vi "UpdateData.vi"(6 "Products":string[](array[string]), 8 "error in (no error)":errorcluster, 9 "Prices":dbl[](array[numeric]), 10 "Stock":i32[](array[numeric]), 11 "Prooduct Actor in":refnum<class "Prooduct Actor.lvclass">) -> (0 "error out":errorcluster, 3 "Prooduct Actor out":refnum<class "Prooduct Actor.lvclass">)   [LabVIEW 2020, in "Prooduct Actor.lvlib" / "Prooduct Actor.lvclass"]
uses:
  Prooduct Actor.lvclass
  Prooduct Actor.lvclass/Prooduct Actor.ctl
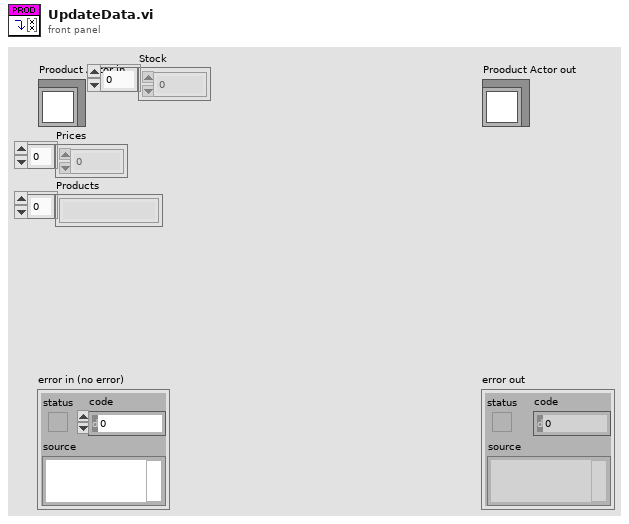
[diagram p1: front panel]
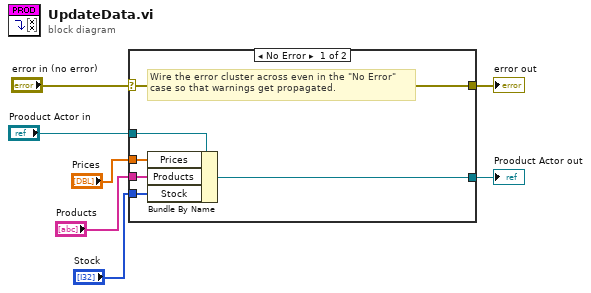
[diagram p0: block diagram]
diagram:
  n1 = case shown="No Error" "error in (no error)" {
    selector: "error in (no error)" -> [w13 w15]
    tunnel: [w13 w15] -> w6
    tunnel: [w11 w14] -> w4
    tunnel: "Prooduct Actor in" -> [w12 w14]
    tunnel: "Stock" -> [w10 _]
    tunnel: "Products" -> [w9 _]
    tunnel: "Prices" -> [w8 _]
    frame No Error {
      # "Wire the error cluster across even in the \"No Error\"\ncase so that warnings get propagated."
      n2 = Bundle By Name(cluster=w12, "Prices"=w8, "Products"=w9, "Stock"=w10) -> (w11:refnum<class "Prooduct Actor.lvclass">)
    }
    frame Error {
    }
  }
  "error out" <- w6
  "Prooduct Actor out" <- w4
